vi "NumberPad.vi"(6 "device ID":refnum<k1>, 7 "Window_Title":string="Numeric Keypad", 8 "Decimals (0)":u8 max=8, 9 "Max_Value (100)":dbl=100.0, 10 "Min_Value (0)":dbl, 11 "Default_Value (0)":dbl) -> (3 "Return_Value":dbl format="%#_8f")   [LabVIEW 2016]
doc: "This VI displays a number pad for user entry via touch-screen or mouse.\n\nB.Reddall & R.Gibson 13-Aug-07"
panel:
  out "Previous":string
  in  "BS_btn":bool
  in  "Clear_btn":bool
  in  "Cancel_btn":bool
  in  "OK_btn":bool
  out "Instruct":string="Please enter a number between:\n0.00 and 100.00"
  out "Display_Value":string="0"
  in  "Neg_btn":bool
  in  "Dot_btn":bool
  out "OutofRange":bool
  in  "NumericButtons":T1
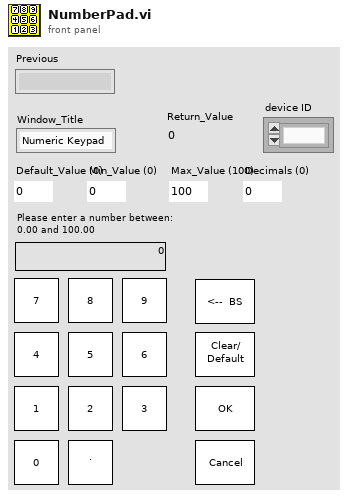
[diagram p1: front panel]
types:
  T1 = cluster{"btn_7":bool, "btn_8":bool, "btn_9":bool, "btn_4":bool, "btn_5":bool, "btn_6":bool, "btn_1":bool, "btn_2":bool, "btn_3":bool, "btn_0":bool}
  T2 = typedef "LVRectTypeDef.ctl" = cluster{"Left":i16, "Top":i16, "Right":i16, "Bottom":i16}
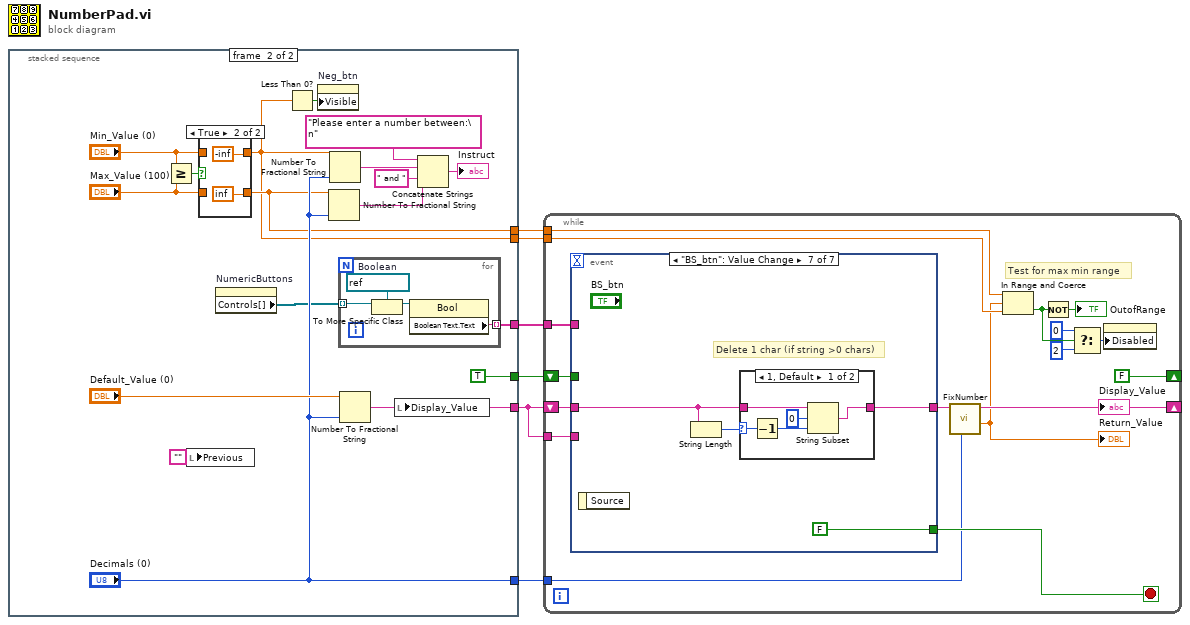
[diagram p0: block diagram]
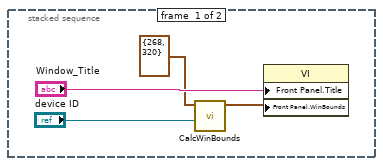
[diagram p2: hidden frame]
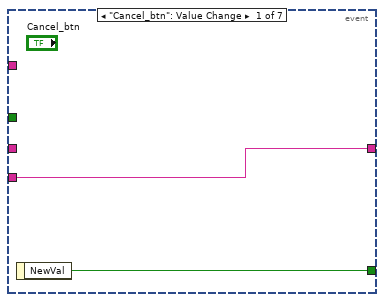
[diagram p4: hidden frame]
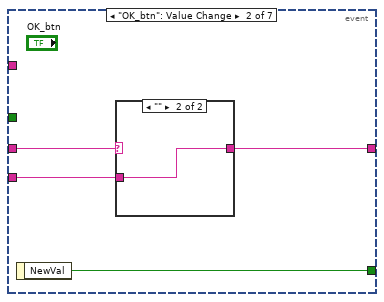
[diagram p5: hidden frame]
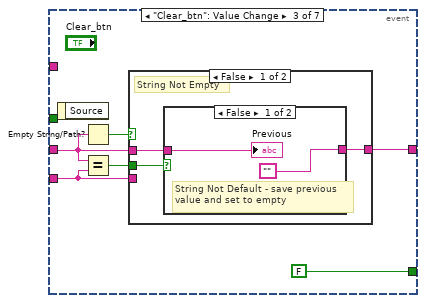
[diagram p7: hidden frame]
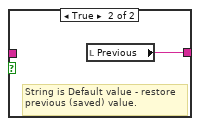
[diagram p8: hidden frame]
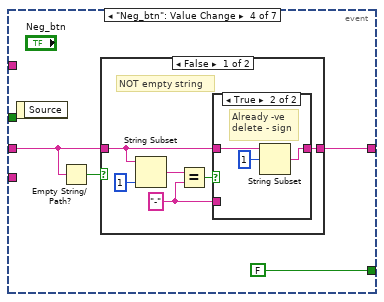
[diagram p10: hidden frame]
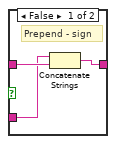
[diagram p11: hidden frame]
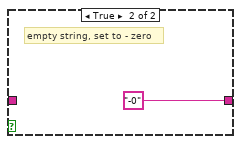
[diagram p12: hidden frame]
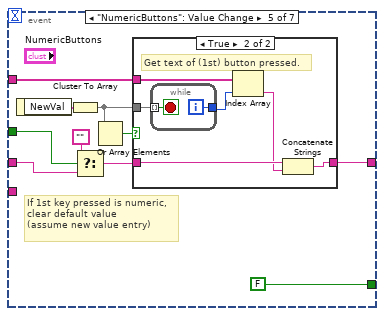
[diagram p13: hidden frame]
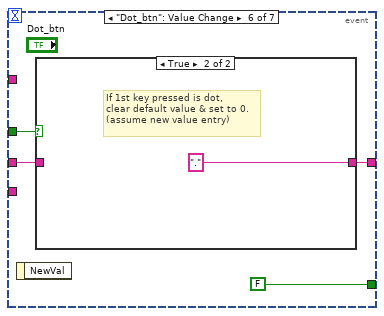
[diagram p15: hidden frame]
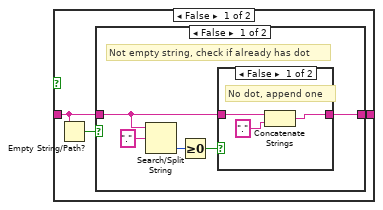
[diagram p16: hidden frame]
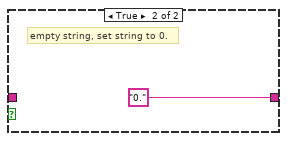
[diagram p18: hidden frame]
diagram:
  n1 = stacked-sequence {
    tunnel: [_ "Decimals (0)"] -> w6
    tunnel: [_ w19] -> w5
    tunnel: [_ w13] -> w4
    tunnel: [_ w14] -> w3
    tunnel: [_ w15] -> w2
    tunnel: [_ TRUE] -> w1
    frame #0 {
      n2 = call "CalcWinBounds.vi"("Mouse device ID"="device ID", "WindowSize"=cluster{"Width":i32, "Height":i32} {"Width"=268, "Height"=320}) -> ("Window Bounds"=w9:T2)  [unwired: 7 out]
      n3 = property class="VI"("Front Panel.Title"="Window_Title", "Front Panel.WinBounds"=w9) -> ()  [unwired: 2 in, 2 out]
    }
    frame #1 {
      n4 = Greater Or Equal?(x="Min_Value (0)", y="Max_Value (100)") -> (x >= y?=w23:bool)
      n5 = local write "Previous"("" ("Previous")) -> ()
      n6 = case shown="True" w23 {
        tunnel: "Min_Value (0)" -> [w34 _]
        tunnel: "Max_Value (100)" -> [w33 _]
        tunnel: [w34 -inf] -> w14
        tunnel: [w33 inf] -> w15
        frame False {
        }
        frame True {
        }
      }
      n7 = property on="NumericButtons" class="Clust"() -> ("Controls[]"=w20:refnum<vi>[])  [unwired: 2 in, 2 out]
      n8 = Less Than 0?(x=w14) -> (x < 0?=w17:bool)
      n9 = property on="Neg_btn" class="Bool"("Visible"=w17) -> ()  [unwired: 2 in, 2 out]
      n10 = Number To Fractional String(number=w15, precision (6)="Decimals (0)") -> (F-format string=w25:string)  [unwired: 2 out]
      n11 = Number To Fractional String(number=w14, precision (6)="Decimals (0)") -> (F-format string=w26:string)  [unwired: 2 out]
      n12 = for {
        tunnel: w20 -> [w32] mode=indexing
        tunnel: [w29] -> w19 mode=indexing
        w30 = refnum<vi> refnum  # Boolean
        n13 = To More Specific Class(target class=w30, reference=w32) -> (specific class reference=w31:refnum<vi>)  [unwired: 1 in, 1 out]
        n14 = property class="Bool"(reference=w31) -> ("Boolean Text.Text"=w29:string)  [unwired: 1 in, 2 out]
      }
      n15 = Number To Fractional String(number="Default_Value (0)", precision (6)="Decimals (0)") -> (F-format string=w13:string)  [unwired: 2 out]
      n16 = local write "Display_Value"(w13) -> ()
      n17 = Concatenate Strings("Please enter a number between:\n" ("string"), w26, " and " ("string"), w25) -> (→"Instruct":string)
    }
  }
  n18 = while {
    shift-right: [w41] -> _
    shift-left: w4 -> [w53]
    tunnel: w6 -> [w40]
    tunnel: w2 -> [w49]
    tunnel: w3 -> [w48]
    tunnel: w5 -> [w51]
    tunnel: w4 -> [w50]
    shift-right: [FALSE] -> _
    shift-left: w1 -> [w37]
    stop <- w52 stop-if-true
    # "Test for max min range"
    n19 = event shown="[6] \"BS_btn\": Value Change" {
      selector: _ -> [_ _ _ _ _ _ _]
      dyn-events: _ -> [_ _ _ _ _ _ _]
      timeout: _ -> [_ _ _ _ _ _ _]
      tunnel: w53 -> [_ w58 w63 w76 w95 w114 w131]
      tunnel: [w54 w57 w66 w77 w97 w113 w130] -> w42
      tunnel: [w55 w59 FALSE ("NewVal") FALSE ("NewVal") FALSE FALSE FALSE] -> w52
      tunnel: w51 -> [_ _ _ _ w98 _ _]
      tunnel: w50 -> [w54 w56 w64 _ _ _ _]
      tunnel: w37 -> [_ _ _ _ w92 w111 _]
      event "Cancel_btn": Value Change {
        n20 = event-data() -> ("NewVal"=w55:bool)  [unwired: 1 out]
      }
      event "OK_btn": Value Change {
        n21 = event-data() -> ("NewVal"=w59:bool)  [unwired: 1 out]
        n22 = case shown="\"\"" w58 {
          selector: w58 -> [w60 _]
          tunnel: [w60 w61] -> w57
          tunnel: w56 -> [_ w61]
          frame "1", Default {
          }
          frame "" {
          }
        }
      }
      event "Clear_btn": Value Change {
        n23 = event-data() -> ()  [unwired: 2 out]
        n24 = Empty String/Path?(string/path=w63) -> (empty?=w65:bool)
        n25 = Equal?(x=w63, y=w64) -> (x = y?=w62:bool)
        n26 = case shown="False" w65 {
          tunnel: [w70 w74] -> w66
          tunnel: w64 -> [_ w74]
          tunnel: w63 -> [w68 _]
          tunnel: w62 -> [w69 _]
          frame False {
            # "String Not Empty"
            n27 = case shown="False" w69 {
              tunnel: ["" w73] -> w70
              tunnel: w68 -> [w72 _]
              frame False {
                # "String Not Default - save previous\nvalue and set to empty"
                "Previous" <- w72
              }
              frame True {
                # "String is Default value - restore\nprevious (saved) value."
                n28 = local read "Previous"() -> (w73:string)
              }
            }
          }
          frame True {
            # "String Empty\n - set to default"
          }
        }
      }
      event "Neg_btn": Value Change {
        n29 = event-data() -> ()  [unwired: 2 out]
        n30 = Empty String/Path?(string/path=w76) -> (empty?=w75:bool)
        n31 = case shown="False" w75 {
          tunnel: w76 -> [w81 _]
          tunnel: [w79 "-0"] -> w77
          frame False {
            w80 = "-"
            # "NOT empty string"
            n32 = String Subset(string=w81, length (rest)=1 ("length (rest)")) -> (substring=w83:string)  [unwired: 1 out]
            n33 = Equal?(x=w83, y=w80) -> (x = y?=w82:bool)
            n34 = case shown="True" w82 {
              tunnel: w81 -> [w86 w90]
              tunnel: [w87 w88] -> w79
              tunnel: w80 -> [w85 _]
              frame False {
                # "Prepend - sign"
                n35 = Concatenate Strings(w85, w86) -> (w87:string)
              }
              frame True {
                # "Already -ve\ndelete - sign"
                n36 = String Subset(string=w90, offset (0)=1) -> (substring=w88:string)  [unwired: 1 out]
              }
            }
          }
          frame True {
            # "empty string, set to - zero"
          }
        }
      }
      event "NumericButtons": Value Change {
        # "If 1st key pressed is numeric,\nclear default value\n(assume new value entry)"
        n37 = event-data() -> ("NewVal"=w101:T1)  [unwired: 1 out]
        n38 = Cluster To Array(cluster=w101) -> (array=w100:bool[])
        n39 = Select(t="", s=w92, f=w95) -> (s? t:f=w94:string)
        n40 = Or Array Elements(Boolean array=w100) -> (logical OR=w99:bool)
        n41 = case shown="True" w99 {
          tunnel: w100 -> [_ w108]
          tunnel: w98 -> [_ w106]
          tunnel: w94 -> [w102 w105]
          tunnel: [w102 w103] -> w97
          frame False {
            # "button released case - do nothing"
          }
          frame True {
            # "Get text of (1st) button pressed."
            n42 = while {
              tunnel: w108 -> [w110] mode=indexing
              tunnel: [w109] -> w107
              i -> [w109]
              stop <- w110 stop-if-true
            }
            n43 = Index Array(array=w106, index=w107) -> (element=w104:string)
            n44 = Concatenate Strings(w105, w104) -> (w103:string)
          }
        }
      }
      event "Dot_btn": Value Change {
        n45 = event-data() -> ()  [unwired: 2 out]
        n46 = case shown="True" w111 {
          tunnel: w114 -> [w117 _]
          tunnel: [w116 "." ("y")] -> w113
          frame False {
            n47 = Empty String/Path?(string/path=w117) -> (empty?=w115:bool)
            n48 = case shown="False" w115 {
              tunnel: w117 -> [w119 _]
              tunnel: [w118 "0." ("y")] -> w116
              frame False {
                # "Not empty string, check if already has dot"
                n49 = Search/Split String(string=w119, search string/char (-)=".") -> (offset of match=w121:i32)  [unwired: 3 out]
                n50 = Greater Or Equal To 0?(x=w121) -> (x >= 0?=w120:bool)
                n51 = case shown="False" w120 {
                  tunnel: [w123 w126] -> w118
                  tunnel: w119 -> [w125 w126]
                  frame False {
                    # "No dot, append one"
                    n52 = Concatenate Strings(w125, "." ("search string/char (-)")) -> (w123:string)
                  }
                  frame True {
                    # "Dot found,\ndo nothing"
                  }
                }
              }
              frame True {
                # "empty string, set string to 0."
              }
            }
          }
          frame True {
            # "If 1st key pressed is dot,\nclear default value & set to 0.\n(assume new value entry)"
          }
        }
      }
      event "BS_btn": Value Change {
        # "Delete 1 char (if string >0 chars)"
        n53 = event-data() -> ()  [unwired: 2 out]
        n54 = String Length(string=w131) -> (length=w132:i32)
        n55 = case shown="1, Default" w132 {
          selector: w132 -> [w137 _]
          tunnel: w131 -> [w134 w138]
          tunnel: [w133 w138] -> w130
          frame 1, Default {
            n56 = Decrement(x=w137) -> (x-1=w135:i32)
            n57 = String Subset(string=w134, offset (0)=0, length (rest)=w135) -> (substring=w133:string)
          }
          frame 0 {
          }
        }
      }
    }
    n58 = call "FixNumber.vi"("Decimals"=w40, "String in"=w42) -> ("value"=w39:dbl, "String out"=w41:string)  [unwired: 6 out]
    "Display_Value" <- w41
    "Return_Value" <- w39
    n59 = In Range and Coerce(upper limit=w49, x=w39, lower limit=w48) -> (In Range?=w45:bool)  [unwired: 1 out]
    n60 = Not(x=w45) -> (.not. x?=→"OutofRange":bool)
    n61 = Select(t=i16 0 ("y"), s=w45, f=i16 2 ("y")) -> (s? t:f=w46:i16)
    n62 = property on="OK_btn" class="Bool"("Disabled"=w46) -> ()  [unwired: 2 in, 2 out]
  }
